vi "Set display mode.vi"(8 "error in (no error)":errorcluster, 10 "Display Mode (def: Hold)":T1=enum."Hold", 11 "VISA resource name":refnum<visa-resource-name>) -> (0 "error out":errorcluster, 3 "VISA resource name out":refnum<visa-resource-name>)   [LabVIEW 2015, in "SR400.lvlib"]
doc: "SD { j }\nIf j = 1, the SD command sets the count display\nmode to HOLD. If j = 0, the display mode will be\nCONTINUOUS. If j is absent, the display mode is\nreturned."
uses:
  SR400.lvlib
  Typedefs/Display Mode.ctl
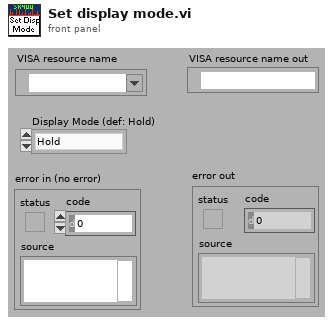
[diagram p1: front panel]
types:
  T1 = typedef "SR400.lvlib/Display Mode.ctl" = enum16{"Continuous", "Hold"}
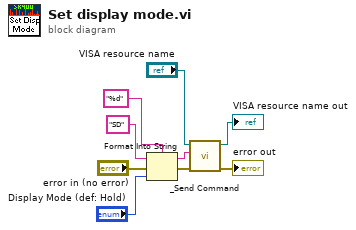
[diagram p0: block diagram]
diagram:
  n1 = Format Into String(format string="%d", initial string="SD" ("command"), error in="error in (no error)", "Display Mode (def: Hold)") -> (resulting string=w5:string, error out=w4:errorcluster)
  n2 = call "_Send Command.vi"("error in (no error)"=w4, "Command"=w5, "VISA resource name"="VISA resource name") -> ("error out"=→"error out":errorcluster, "VISA resource name out"=→"VISA resource name out":refnum<visa-resource-name>)  [unwired: 1 in, 6 out]
